vi "FDMR+ read TDMS properties.vi"(8 "error in (no error)":errorcluster, 10 "cahnnel group name in":string, 11 "TDMS ref in":refnum<k34>) -> (0 "error out":errorcluster, 1 "group name out":string, 2 "FDMR+ measurement parameters":T1={"F_start [GHz]"=0.0, "F_end [GHz]"=0.0, "Field [T]"=0.0, "Points [-]"=0, "Sampling Rate"=15, "ModA [G]"=0.0, "ModF [kHz]"=0.0, "Time const [ms]"=0.0, "Angle [°]"=0.0, "Tmp [K]"=0.0, "Wait [min]"=0.0, "Repeat [-]"=0, "Comment"="", "Execute"=FALSE, "Auto-mod"=FALSE} {"Sampling Rate" items=["117 ks/S"=9, "58.6 kS/s"=10, "29.3 kS/s"=11, "14.6 kS/s"=12, "7.32 kS/s"=13, "3.66 kS/s"=14, "1.83 kS/s"=15]; "Time const [ms]" min=-1.0 max=330.0; "ModF [kHz]" min=0.2 max=120.0; "Repeat [-]" max=1048576; "Points [-]" max=50; "Wait [min]" max=1048576.0; "Field [T]" min=-16.0 max=16.0}, 3 "TDMS ref out":refnum<k34>)   [LabVIEW 2024]
uses:
  Datatypes/FDMR+ script line.ctl
  Subsystem modules/Lock-in module/ctl/OSC sampling rate.ctl
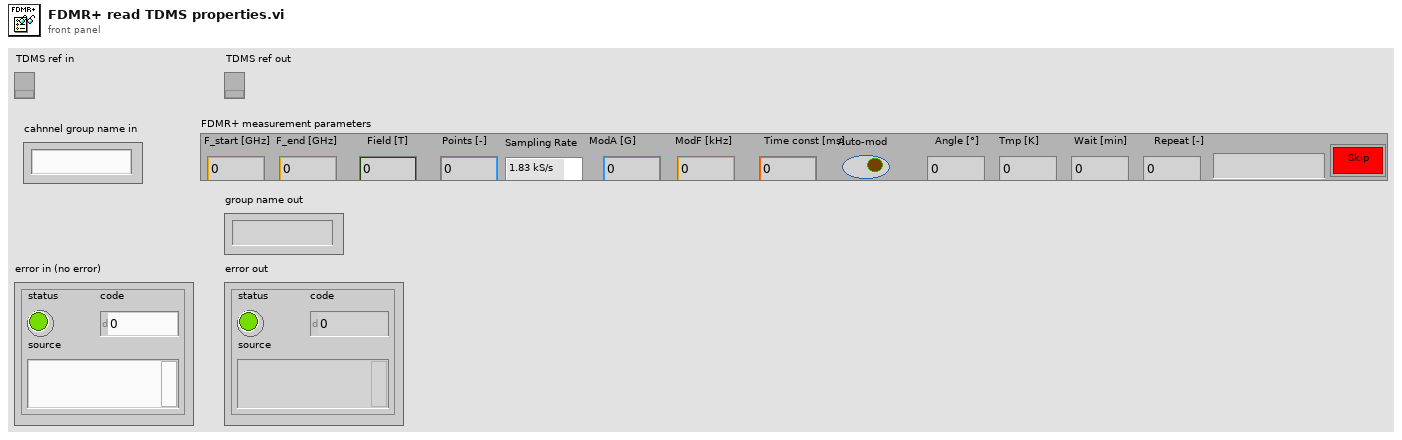
[diagram p1: front panel]
types:
  T1 = typedef "FDMR+ script line.ctl" = cluster{"F_start [GHz]":dbl, "F_end [GHz]":dbl, "Field [T]":dbl, "Points [-]":u32, "Sampling Rate":T2, "ModA [G]":dbl, "ModF [kHz]":dbl, "Time const [ms]":dbl, "Angle [°]":dbl, "Tmp [K]":dbl, "Wait [min]":dbl, "Repeat [-]":i32, "Comment":string, "Execute":bool, "Auto-mod":bool}
  T2 = typedef "OSC sampling rate.ctl" = u16
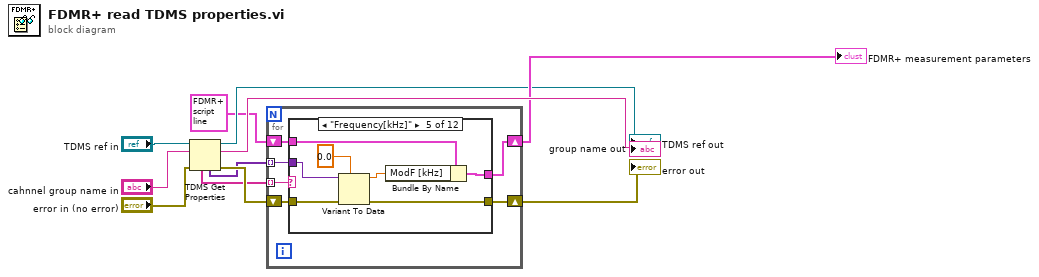
[diagram p0: block diagram]
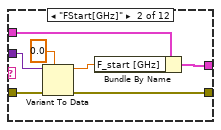
[diagram p3: hidden frame]
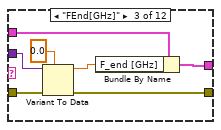
[diagram p4: hidden frame]
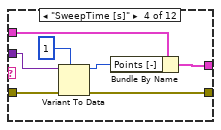
[diagram p5: hidden frame]
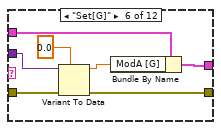
[diagram p6: hidden frame]
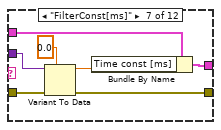
[diagram p7: hidden frame]
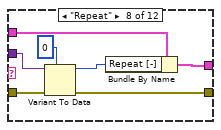
[diagram p8: hidden frame]
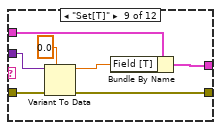
[diagram p9: hidden frame]
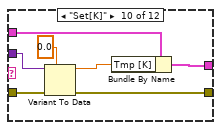
[diagram p10: hidden frame]
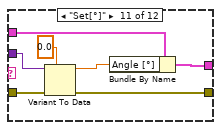
[diagram p11: hidden frame]
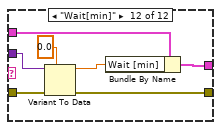
[diagram p12: hidden frame]
diagram:
  n1 = TDMS Get Properties(8:"error in (no error)", 10:"cahnnel group name in", 11:"TDMS ref in") -> (0:w4:errorcluster, 2:→"group name out":string, 3:→"TDMS ref out":refnum<k34>, 4:w2:variant[], 6:w1:string[])  [unwired: 3 in, 1 out]
  n2 = for {
    tunnel: w2 -> [w17] mode=indexing
    tunnel: w1 -> [w16] mode=indexing
    shift-right: [w14] -> w9
    shift-left: T1 {"F_start [GHz]"=380.0, "F_end [GHz]"=400.0, "Field [T]"=0.0, "Points [-]"=1, "Sampling Rate"=15, "ModA [G]"=1.0, "ModF [kHz]"=10.0, "Time const [ms]"=1.0, "Angle [°]"=-1.0, "Tmp [K]"=295.0, "Wait [min]"=0.0, "Repeat [-]"=0, "Comment"="", "Execute"=FALSE, "Auto-mod"=FALSE} ("FDMR+ script line") -> [w15]
    shift-right: [w12] -> w8
    shift-left: w4 -> [w13]
    n3 = case shown="\"Frequency[kHz]\"" w16 {
      tunnel: w17 -> [_ w24 w31 w38 w45 w52 w59 w66 w73 w80 w87 w94]
      tunnel: w15 -> [w19 w26 w33 w40 w47 w54 w61 w68 w75 w82 w89 w96]
      tunnel: [w19 w25 w32 w39 w46 w53 w60 w67 w74 w81 w88 w95] -> w14
      tunnel: w13 -> [w18 w21 w28 w37 w44 w51 w58 w65 w72 w79 w86 w93]
      tunnel: [w18 w20 w27 w36 w43 w50 w57 w64 w71 w78 w85 w92] -> w12
      frame Default {
      }
      frame "FStart[GHz]" {
        n4 = Variant To Data(error in=w21, type=0.0 ("F_start [GHz]"), Variant=w24) -> (data=w22:dbl, error out=w20:errorcluster)
        n5 = Bundle By Name(cluster=w26, "F_start [GHz]"=w22) -> (w25:T1)
      }
      frame "FEnd[GHz]" {
        n6 = Variant To Data(error in=w28, type=0.0 ("F_start [GHz]"), Variant=w31) -> (data=w29:dbl, error out=w27:errorcluster)
        n7 = Bundle By Name(cluster=w33, "F_end [GHz]"=w29) -> (w32:T1)
      }
      frame "SweepTime [s]" {
        n8 = Variant To Data(error in=w37, type=u32 1, Variant=w38) -> (data=w34:u32, error out=w36:errorcluster)
        n9 = Bundle By Name(cluster=w40, "Points [-]"=w34) -> (w39:T1)
      }
      frame "Frequency[kHz]" {
        n10 = Variant To Data(error in=w44, type=0.0, Variant=w45) -> (data=w42:dbl, error out=w43:errorcluster)
        n11 = Bundle By Name(cluster=w47, "ModF [kHz]"=w42) -> (w46:T1)
      }
      frame "Set[G]" {
        n12 = Variant To Data(error in=w51, type=0.0, Variant=w52) -> (data=w49:dbl, error out=w50:errorcluster)
        n13 = Bundle By Name(cluster=w54, "ModA [G]"=w49) -> (w53:T1)
      }
      frame "FilterConst[ms]" {
        n14 = Variant To Data(error in=w58, type=0.0, Variant=w59) -> (data=w56:dbl, error out=w57:errorcluster)
        n15 = Bundle By Name(cluster=w61, "Time const [ms]"=w56) -> (w60:T1)
      }
      frame "Repeat" {
        n16 = Variant To Data(error in=w65, type=u32 0, Variant=w66) -> (data=w63:u32, error out=w64:errorcluster)
        n17 = Bundle By Name(cluster=w68, "Repeat [-]"=w63) -> (w67:T1)
      }
      frame "Set[T]" {
        n18 = Variant To Data(error in=w72, type=0.0, Variant=w73) -> (data=w70:dbl, error out=w71:errorcluster)
        n19 = Bundle By Name(cluster=w75, "Field [T]"=w70) -> (w74:T1)
      }
      frame "Set[K]" {
        n20 = Variant To Data(error in=w79, type=0.0, Variant=w80) -> (data=w77:dbl, error out=w78:errorcluster)
        n21 = Bundle By Name(cluster=w82, "Tmp [K]"=w77) -> (w81:T1)
      }
      frame "Set[°]" {
        n22 = Variant To Data(error in=w86, type=0.0, Variant=w87) -> (data=w84:dbl, error out=w85:errorcluster)
        n23 = Bundle By Name(cluster=w89, "Angle [°]"=w84) -> (w88:T1)
      }
      frame "Wait[min]" {
        n24 = Variant To Data(error in=w93, type=0.0, Variant=w94) -> (data=w91:dbl, error out=w92:errorcluster)
        n25 = Bundle By Name(cluster=w96, "Wait [min]"=w91) -> (w95:T1)
      }
    }
  }
  "FDMR+ measurement parameters" <- w9
  "error out" <- w8
